vi "light_decoupling.vi"(6 "Reset":bool, 10 "Configuration":T1, 11 "Array in":sgl[][](array[numeric])=[[0.0, 0.0, 0.0, 0.0]]) -> (3 "Array out":sgl[][](array[numeric]))   [LabVIEW 2013]
uses:
  initialization/configuration.ctl
  initialization/asap_calibration.ctl
  <vilib>/Analysis/Matrix/Datatypes/RealMatrix.ctl
  utilities/labview/norm_vec_single.vi
  <vilib>/Analysis/Matrix/NI_Matrix.lvlib
panel:
  in  "Calibration slope":sgl=0.00020504874 format="%#_3p"
  out "Adjustment":sgl[][](array[numeric])
  in  "Enable":bool
  # "Each row is the normalized axis positions for one light."
  # "Axis position coupling vs 1/distance, in normalized axis position units."
  # "Call at least once with Reset true\nto cache the LUT."
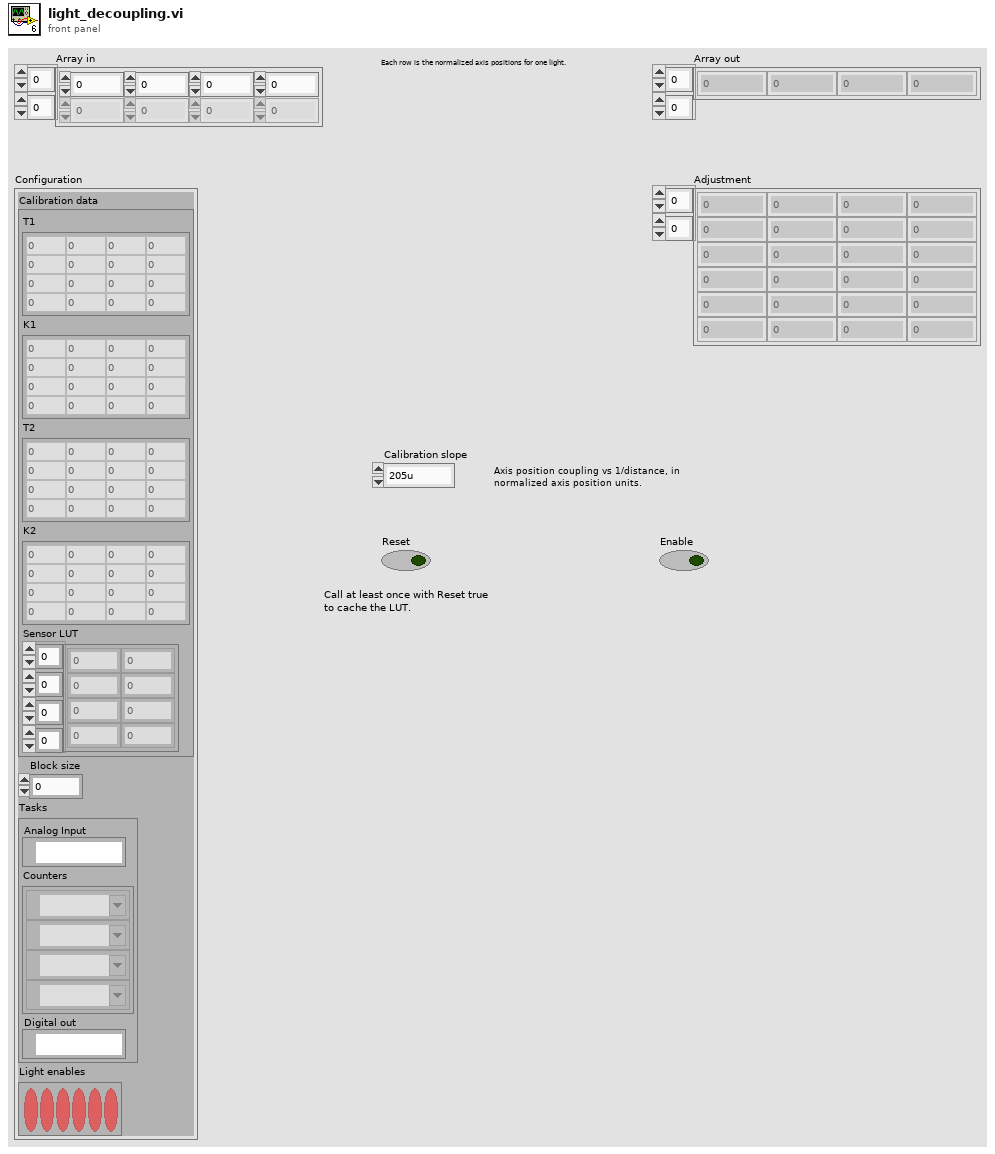
[diagram p1: front panel]
types:
  T1 = typedef "configuration.ctl" = cluster{"Calibration data":T2, "Block size":i32, "Tasks":cluster{"Analog Input":refnum<k21>, "Counters":refnum<k21>[], "Digital out":refnum<k21>}, "Light enables":bool[]}
  T2 = typedef "asap_calibration.ctl" = cluster{"T1":T3, "K1":T3, "T2":T3, "K2":T3, "Sensor LUT":sgl[][][][]}
  T3 = typedef "NI_Matrix.lvlib/RealMatrix.ctl" = dbl[][]
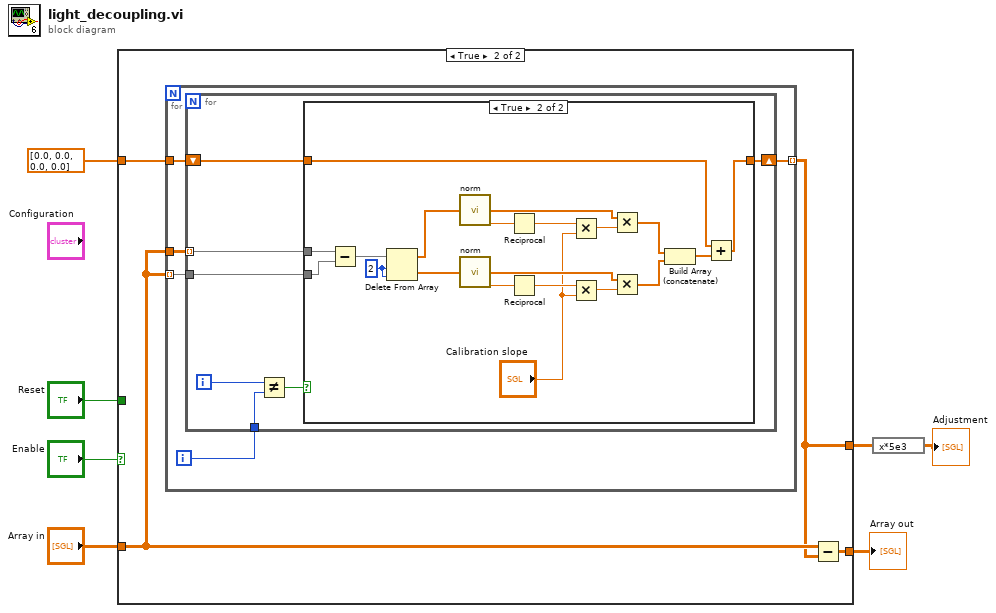
[diagram p0: block diagram]
diagram:
  n1 = case shown="True" "Enable" {
    tunnel: "Reset" -> [_ _]
    tunnel: [w8 w12] -> w5
    tunnel: "Array in" -> [w8 w11]
    tunnel: [w8 w9] -> w6
    tunnel: sgl[] [0.0, 0.0, 0.0, 0.0] ("array w/ subset deleted") -> [_ w10]
    frame False {
    }
    frame True {
      n2 = for {
        tunnel: w11 -> [w16] mode=indexing
        tunnel: w11 -> [w17]
        tunnel: [w15] -> w9 mode=indexing
        tunnel: w10 -> [w14]
        i -> [w13]
        n3 = for {
          tunnel: w17 -> [w24] mode=indexing
          tunnel: w16 -> [w23]
          shift-right: [w22] -> w15
          shift-left: w14 -> [w21]
          tunnel: w13 -> [w19]
          i -> [w20]
          n4 = Not Equal?(x=w20, y=w19) -> (x != y?=w18:bool)
          n5 = case shown="True" w18 {
            tunnel: w24 -> [_ w45]
            tunnel: w23 -> [_ w44]
            tunnel: [w25 w27] -> w22
            tunnel: w21 -> [w25 w26]
            frame False {
            }
            frame True {
              w43 = 2 ("length")
              n6 = Subtract(x=w45, y=w44) -> (x-y=w42:sgl[])
              n7 = Delete From Array(array=w42, length=w43, index=w43) -> (deleted portion=w32:sgl[], array with subset deleted=w41:sgl[])
              n8 = call-poly "norm.vi"("vector"=w41) -> ("magnitude"=w40:sgl, "normalized vector"=w37:sgl[])  [unwired: 3 in]
              n9 = call-poly "norm.vi"("vector"=w32) -> ("magnitude"=w33:sgl, "normalized vector"=w36:sgl[])  [unwired: 3 in]
              n10 = Reciprocal(x=w40) -> (1/x=w39:sgl)
              n11 = Reciprocal(x=w33) -> (1/x=w34:sgl)
              n12 = Multiply(x=w39, y="Calibration slope") -> (x*y=w38:sgl)
              n13 = Multiply(x=w34, y="Calibration slope") -> (x*y=w35:sgl)
              n14 = Multiply(x=w37, y=w38) -> (x*y=w30:sgl[])
              n15 = Multiply ("Multiply.vi")(x=w36, y=w35) -> (x*y=w29:sgl[])
              n16 = Build Array (concatenate)(w30, w29) -> (w28:sgl[])
              n17 = Add(x=w26, y=w28) -> (x+y=w27:sgl[])
            }
          }
        }
      }
      n18 = Subtract(x=w11, y=w9) -> (x-y=w12:sgl[][])
    }
  }
  "Array out" <- w5
  n19 = expression code="x*5e3"(w6) -> (→"Adjustment":sgl[][])
